vi "Setup.vi"(8 "Error In":errorcluster, 9 "Password":string, 10 "Username":string, 11 "Address":string) -> (0 "Error Out":errorcluster, 3 "Listener":refnum<class "Listener.lvclass">)   [LabVIEW 2018, in "Tests.lvlib" / "Listener.lvlib"]
uses:
  Listener.lvlib
  src/Toolkit/Listener/Listener.lvclass
  src/Toolkit/Session/Support/Password Authentication.vi
  src/Toolkit/Listener/Support/Create from Session.vi
  src/Toolkit/SSH/SSH.lvclass
  src/Toolkit/Session/Session.lvclass
  Tests.lvlib
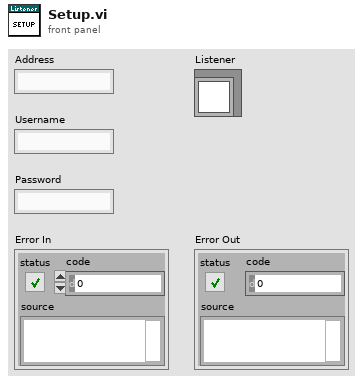
[diagram p1: front panel]
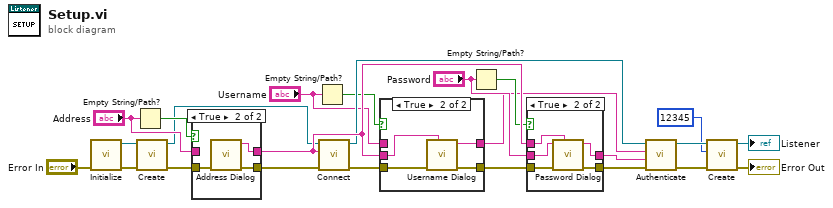
[diagram p0: block diagram]
diagram:
  n1 = call "Initialize.vi"("Error In"="Error In") -> ("Error Out"=w6:errorcluster, "SSH"=w7:refnum<class "SSH.lvclass">)  [unwired: 9 in]
  n2 = Empty String/Path?(string/path="Address") -> (empty?=w10:bool)
  n3 = call "Create.vi"("Error In"=w6, "SSH"=w7) -> ("Error Out"=w12:errorcluster, "Sesssion"=w9:refnum<class "Session.lvclass">)  [unwired: 8 in]
  n4 = case shown="True" w10 {
    tunnel: w12 -> [w25 w29]
    tunnel: [w25 w28] -> w13
    tunnel: [w26 w27] -> w24
    tunnel: "Address" -> [w26 _]
    frame False {
    }
    frame True {
      n5 = call "Address Dialog.vi"("Error In"=w29) -> ("Error Out"=w28:errorcluster, "Address Out"=w27:string)  [unwired: 9 in]
    }
  }
  n6 = Empty String/Path?(string/path="Username") -> (empty?=w19:bool)
  n7 = call "Connect.vi"("Error In"=w13, "Address"=w24, "Session In"=w9) -> ("Error Out"=w22:errorcluster, "Sesssion Out"=w23:refnum<class "Session.lvclass">)  [unwired: 7 in]
  n8 = case shown="True" w19 {
    tunnel: w22 -> [w31 w35]
    tunnel: [w30 w34] -> w17
    tunnel: [w31 w33] -> w14
    tunnel: "Username" -> [w30 _]
    tunnel: w24 -> [_ w32]
    frame False {
    }
    frame True {
      n9 = call "Username Dialog.vi"("Address"=w32, "Error In"=w35) -> ("Error Out"=w33:errorcluster, "Username Out"=w34:string)  [unwired: 8 in]
    }
  }
  n10 = Empty String/Path?(string/path="Password") -> (empty?=w21:bool)
  n11 = case shown="True" w21 {
    tunnel: "Password" -> [w37 w42]
    tunnel: w14 -> [w36 w41]
    tunnel: [w36 w40] -> w15
    tunnel: [w37 w39] -> w16
    tunnel: w24 -> [_ w38]
    frame False {
    }
    frame True {
      n12 = call "Password Dialog.vi"("Address"=w38, "Error In"=w41, "Password In"=w42) -> ("Error Out"=w40:errorcluster, "Password Out"=w39:string)  [unwired: 7 in]
    }
  }
  n13 = call-poly "Authenticate.vi"("Error In"=w15, "Password"=w16, "Username"=w17, "Session In"=w23) -> ("Error Out"=w4:errorcluster, "Sesssion Out"=w5:refnum<class "Session.lvclass">)  [unwired: 6 in]
  n14 = call-poly "Create.vi"("Error In"=w4, "Port"=12345, "Session"=w5) -> ("Error Out"=→"Error Out":errorcluster, "Listener"=→"Listener":refnum<class "Listener.lvclass">)  [unwired: 7 in]
